vi "Read Tokens.vi"(8 "error in (no error)":errorcluster, 11 "input string":string) -> (0 "error out":errorcluster, 2 "Token Secret":string, 3 "Token":string)   [LabVIEW 2011, in "i3-oauth.lvlib"]
uses:
  i3-oauth.lvlib
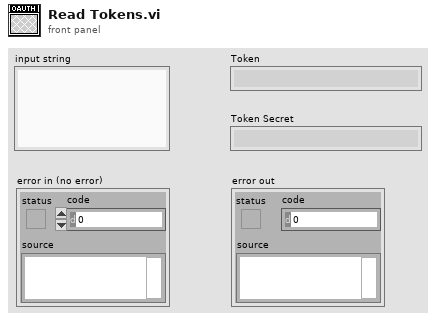
[diagram p1: front panel]
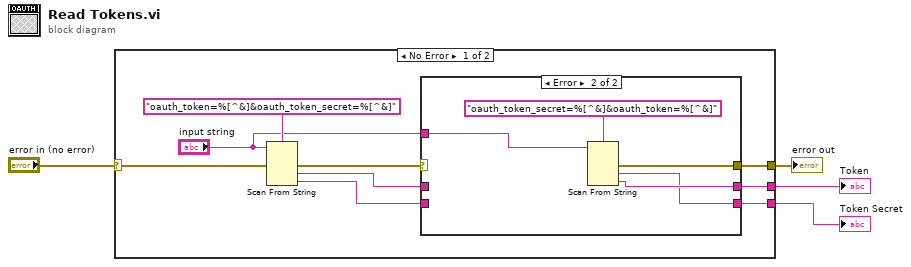
[diagram p0: block diagram]
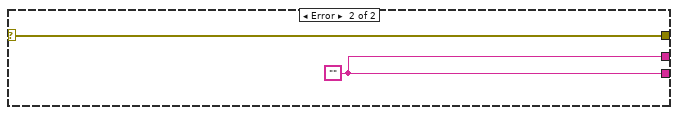
[diagram p3: hidden frame]
diagram:
  n1 = case shown="No Error" "error in (no error)" {
    selector: "error in (no error)" -> [w8 w23]
    tunnel: [w9 w23] -> w4
    tunnel: [w7 w22] -> w2
    tunnel: [w6 w22] -> w1
    frame No Error {
      n2 = Scan From String(format string="oauth_token=%[^&]&oauth_token_secret=%[^&]", input string="input string", error in=w8) -> (error out=w12:errorcluster, output 1=w11:string, output 2=w10:string)  [unwired: 3 in, 2 out]
      n3 = case shown="Error" w12 {
        selector: w12 -> [w14 _]
        tunnel: "input string" -> [_ w20]
        tunnel: w11 -> [w15 _]
        tunnel: w10 -> [w16 _]
        tunnel: [w16 w18] -> w6
        tunnel: [w15 w19] -> w7
        tunnel: [w14 w17] -> w9
        frame No Error {
        }
        frame Error {
          n4 = Scan From String(format string="oauth_token_secret=%[^&]&oauth_token=%[^&]", input string=w20) -> (error out=w17:errorcluster, output 1=w18:string, output 2=w19:string)  [unwired: 4 in, 2 out]
        }
      }
    }
    frame Error {
      w22 = ""
    }
  }
  "error out" <- w4
  "Token" <- w2
  "Token Secret" <- w1
